vi "bk9132b Set_Chxx.vi"(6 "Enable Output":bool, 7 "Chanel (1-3)":u8, 9 "Current":dbl format="%.2f", 10 "Voltage":dbl format="%.2g", 11 "VISA resource name":refnum<visa-resource-name>) -> (0 "error out":errorcluster)   [LabVIEW 2018]
uses:
  <instrlib>/BK Precision 913XX/BK Precision 913XX.lvlib
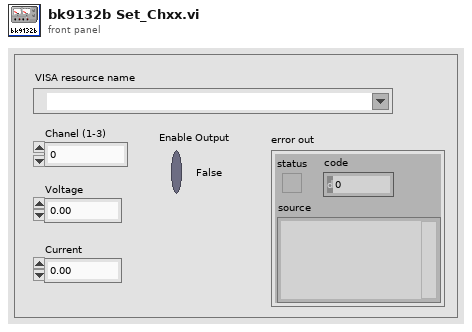
[diagram p1: front panel]
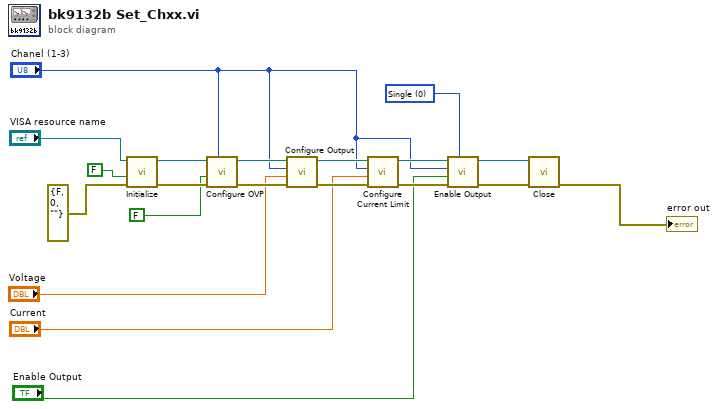
[diagram p0: block diagram]
diagram:
  w6 = u16 0 items=["Single", "All"] ("Control Mode (0:Single)")
  n1 = call <instrlib>:"Initialize.vi"("error in (no error)"=errorcluster {"status"=FALSE, "code"=0, "source"=""}, "Reset (True)"=FALSE, "VISA resource name"="VISA resource name") -> ("error out"=w17:errorcluster, "VISA resource name out"=w12:refnum<visa-resource-name>)  [unwired: 7 in]
  n2 = call <instrlib>:"Configure OVP.vi"("Channel (1:1)"="Chanel (1-3)", "error in (no error)"=w17, "Enable OVP (T: Enable)"=FALSE, "VISA resource name"=w12) -> ("error out"=w16:errorcluster, "VISA resource name out"=w11:refnum<visa-resource-name>)  [unwired: 6 in]
  n3 = call <instrlib>:"Configure Output.vi"("error in (no error)"=w16, "Voltage Level (0.0 V)"="Voltage", "Channel (1:1)"="Chanel (1-3)", "VISA resource name"=w11) -> ("error out"=w15:errorcluster, "VISA resource name out"=w10:refnum<visa-resource-name>)  [unwired: 6 in]
  n4 = call <instrlib>:"Configure Current Limit.vi"("error in (no error)"=w15, "Current Limit (0.0 A)"="Current", "Channel (1:1)"="Chanel (1-3)", "VISA resource name"=w10) -> ("error out"=w14:errorcluster, "VISA resource name out"=w9:refnum<visa-resource-name>)  [unwired: 6 in]
  n5 = call <instrlib>:"Enable Output.vi"("Control Mode (0:Single)"=w6, "error in (no error)"=w14, "Enable Output (F: False)"="Enable Output", "Channel (1:1)"="Chanel (1-3)", "VISA resource name"=w9) -> ("error out"=w13:errorcluster, "VISA resource name out"=w8:refnum<visa-resource-name>)  [unwired: 5 in]
  n6 = call <instrlib>:"Close.vi"("error in (no error)"=w13, "VISA resource name"=w8) -> ("error out"=→"error out":errorcluster)  [unwired: 9 in]
